vi "Async Update.vi"(8 "error in":errorcluster, 10 "Frame Info Array":T3[](array[typedef]), 11 "Interupt Q":refnum<queue>) -> (0 "error out":errorcluster, 1 "timed out?":bool, 2 "Frame Info Array":T3[](array[typedef]), 3 "Stop":bool)   [LabVIEW 2024]
doc: "All Rights Reserved © 2017 SyncSols"
uses:
  Controls/Async Frame Info Cluster.ctl
  Controls/Async Message Info Cluster.ctl
  TCP Engine/Controls/TCP Engine Serial Interupt Cluster.ctl
  Controls/Async Update Cluster.ctl
  TCP Engine/TCP Engine.lvlib
panel:
  in  "value":T1
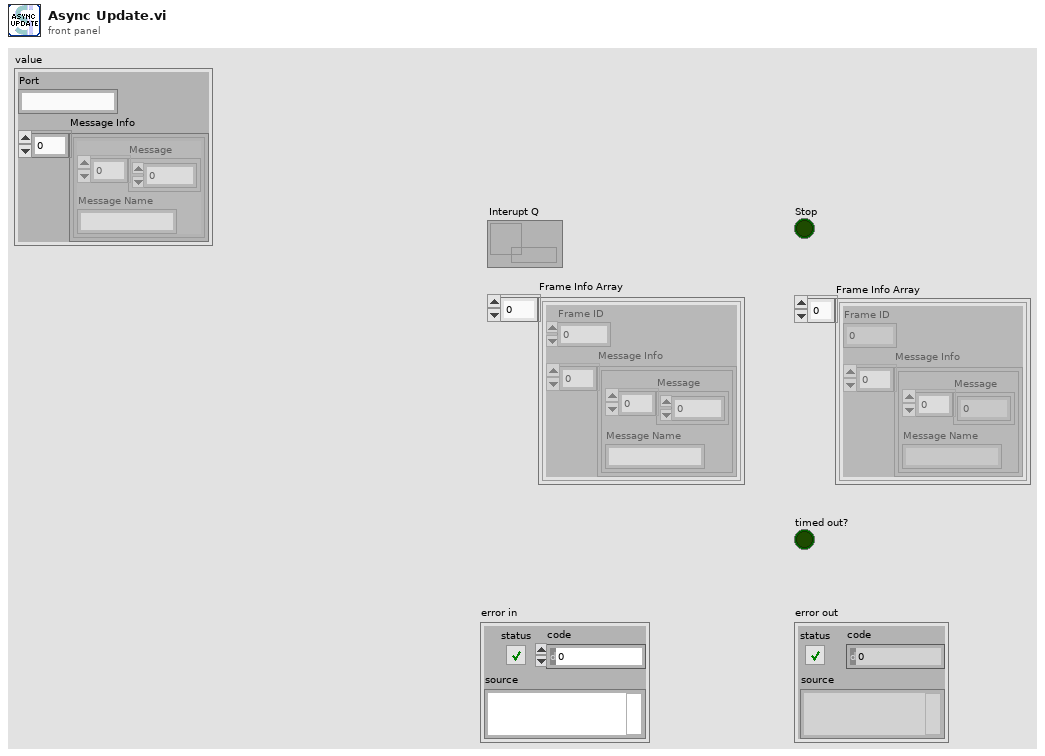
[diagram p1: front panel]
types:
  T1 = typedef "Async Update Cluster.ctl" = cluster{"Port":string, "Message Info":T2[]}
  T2 = typedef "Async Message Info Cluster.ctl" = cluster{"Message":u8[], "Message Name":string}
  T3 = typedef "Async Frame Info Cluster.ctl" = cluster{"Frame ID":u16, "Message Info":T2[]}
  T4 = typedef "TCP Engine.lvlib/TCP Engine Serial Interupt Cluster.ctl" = cluster{"Stop":bool, "JSON Variant":variant}
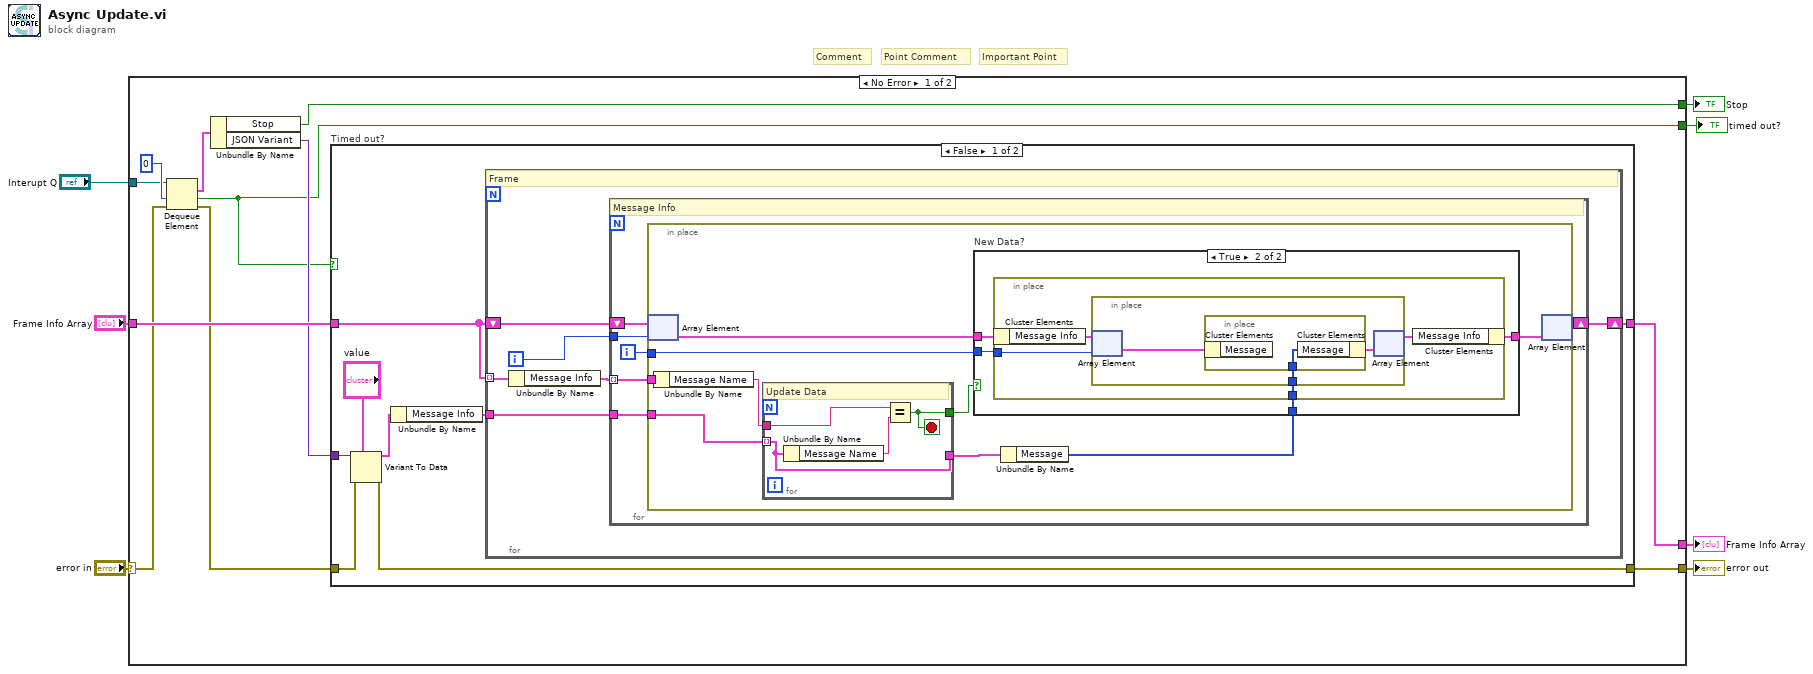
[diagram p0: block diagram]
diagram:
  # "Important Point"
  # "Point Comment"
  # "Comment"
  n1 = case shown="No Error" "error in" {
    selector: "error in" -> [w12 w68]
    tunnel: [w8 w68] -> w7
    tunnel: "Frame Info Array" -> [w16 w67]
    tunnel: "Interupt Q" -> [w15 _]
    tunnel: [w13 _] -> w3
    tunnel: [w10 w67] -> w2
    tunnel: [w9 _] -> w1
    frame No Error {
      n2 = Dequeue Element(queue=w15, timeout in ms (-1)=0, error in (no error)=w12) -> (element=w17:T4, timed out?=w9:bool, error out=w11:errorcluster)  [unwired: 1 out]
      n3 = Unbundle By Name(w17) -> ("Stop"=w13:bool, "JSON Variant"=w14:variant)
      n4 = case "Timed out?" shown="False" w9 {
        tunnel: w14 -> [w26 _]
        tunnel: [w24 w65] -> w8
        tunnel: [w22 w66] -> w10
        tunnel: w16 -> [w21 w66]
        tunnel: w11 -> [w20 w65]
        frame False {
          n5 = Variant To Data(error in=w20, type="value", Variant=w26) -> (data=w25:T1, error out=w24:errorcluster)
          n6 = Unbundle By Name(w25) -> ("Message Info"=w23:T2[])
          n7 = for {
            tunnel: w23 -> [w30]
            tunnel: w21 -> [w32] mode=indexing
            shift-right: [w28] -> w22
            shift-left: w21 -> [w29]
            i -> [w27]
            # "Frame"
            n8 = Unbundle By Name(w32) -> ("Message Info"=w31:T2[])
            n9 = for {
              tunnel: w31 -> [w38] mode=indexing
              tunnel: w30 -> [w37]
              shift-right: [w33] -> w28
              shift-left: w29 -> [w35]
              tunnel: w27 -> [w34]
              i -> [w36]
              # "Message Info"
              n10 = in-place {
                in-place-border: w38 -> [w47]
                in-place-border: w37 -> [w45]
                in-place-border: w36 -> [w44]
                n11 = in-place-array #1(w35, w34) -> (w41:T3)
                n12 = Unbundle By Name(w47) -> ("Message Name"=w46:string)
                n13 = for {
                  tunnel: w46 -> [w63]
                  tunnel: w45 -> [w62] mode=indexing
                  tunnel: [w62] -> w43
                  tunnel: [w61] -> w39
                  stop <- w61 stop-if-true
                  # "Update Data"
                  n14 = Unbundle By Name(w62) -> ("Message Name"=w64:string)
                  n15 = Equal?(x=w63, y=w64) -> (x = y?=w61:bool)
                }
                n16 = Unbundle By Name(w43) -> ("Message"=w42:u8[])
                n17 = case "New Data?" shown="True" w39 {
                  tunnel: w44 -> [_ w52]
                  tunnel: w41 -> [w48 w51]
                  tunnel: w42 -> [_ w50]
                  tunnel: [w48 w49] -> w40
                  frame False {
                  }
                  frame True {
                    n18 = in-place {
                      in-place-border: w52 -> [w56]
                      in-place-border: w50 -> [w54]
                      n19 = in-place-cluster #2(w51) -> ("Message Info"=w55:T2[])
                      n20 = in-place {
                        in-place-border: w54 -> [w58]
                        n21 = in-place-array #3(w55, w56) -> (w59:T2)
                        n22 = in-place {
                          in-place-border: w58 -> [w60]
                          n23 = in-place-cluster #4(w59) -> ()  [unwired: 1 out]
                          n24 = in-place-cluster #4("Message"=w60) -> (w57:T2)
                        }
                        n25 = in-place-array #3(w57) -> (w53:T2[])  [unwired: 1 out]
                      }
                      n26 = in-place-cluster #2("Message Info"=w53) -> (w49:T3)
                    }
                  }
                }
                n27 = in-place-array #1(w40) -> (w33:T3[])  [unwired: 1 out]
              }
            }
          }
        }
        frame True {
        }
      }
    }
    frame Error {
    }
  }
  "error out" <- w7
  "Stop" <- w3
  "Frame Info Array" <- w2
  "timed out?" <- w1
